vi "ScanSystemInfo.vi"(0 "refnum":refnum<file>, 11 "offset":i32) -> (1 "Scan Settings":T1 {"prf (kHz)" format="%.2f"; "GAIN(db)" items=["26.0", "40.0", "54.0"]; "LP FILT(IN MHz)" items=["20", "50", "100", "200"]; "HP FILT(IN KHz)" items=["1", "1000", "3000", "10000"]; "DAMPING (IN Ohm)" items=["7", "10", "16", "20", "26", "30", "40", "50"]; "ENERGY(UJ)" items=["1", "2", "4", "8", "16", "32"]}, 2 "Energy":u8, 3 "Damping":u8, 4 "dup refnum":refnum<file>, 6 "High Pass":u8, 8 "Gain":u8, 10 "prf (kHz)":sgl format="%.2f", 14 "Distance between\nscan planes (mm)":u16, 15 "Distance between\nscan lines (mm)":u16)   [LabVIEW 2022 SP3]
panel:
  out "Low Pass":u8
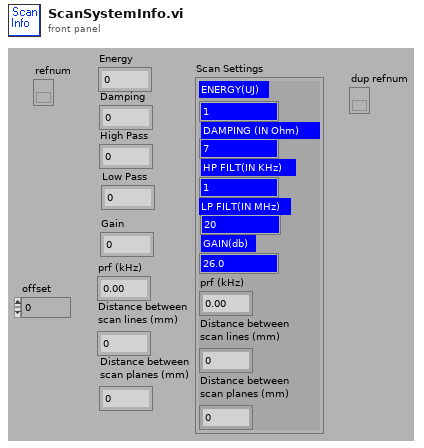
[diagram p1: front panel]
types:
  T1 = cluster{"ENERGY(UJ)":u8, "DAMPING (IN Ohm)":u8, "HP FILT(IN KHz) ":u8, "LP FILT(IN MHz)":u8, "GAIN(db)":u8, "prf (kHz)":sgl, "Distance between\nscan lines (mm)":u16, "Distance between\nscan planes (mm)":u16}
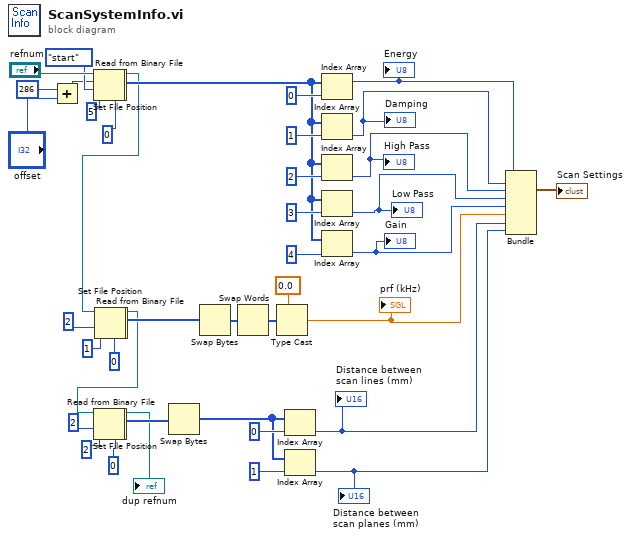
[diagram p0: block diagram]
diagram:
  n1 = Add(x=286 ("pos offset (0)"), y="offset") -> (x+y=w9:i32)
  n2 = Set File Position(offset (in bytes) (0)=w9, refnum="refnum", from (0:start)=enum16{"start", "end", "current"}."start" ("pos mode (0:2)")) -> (refnum out=w2:refnum<file>, error out=w1:errorcluster)  [unwired: 1 in]
  n3 = Read from Binary File(5:u8 0, 8:w1, 10:5 ("count"), 11:w2) -> (2:w26:u8[], 3:w25:refnum<file>)  [unwired: 4 out]
  n4 = Set File Position(refnum=w25, from (0:start)=2) -> (refnum out=w6:refnum<file>, error out=w5:errorcluster)  [unwired: 1 in, 1 out]
  n5 = Read from Binary File(5:0 ("byte stream type"), 8:w5, 10:1 ("count"), 11:w6) -> (2:w29:i32[], 3:w20:refnum<file>)  [unwired: 4 out]
  n6 = Set File Position(refnum=w20, from (0:start)=2) -> (refnum out=w4:refnum<file>, error out=w3:errorcluster)  [unwired: 1 in, 1 out]
  n7 = Read from Binary File(5:u16 0, 8:w3, 10:2 ("count"), 11:w4) -> (2:w17:u16[], 3:→"dup refnum":refnum<file>)  [unwired: 4 out]
  n8 = Swap Bytes(anything=w17) -> (byte swapped=w14:u16[])
  n9 = Swap Bytes(anything=w29) -> (byte swapped=w28:i32[])
  n10 = Swap Words(1:w28) -> (0:w27:i32[])
  n11 = Type Cast(type=sgl 0.0, x=w27) -> (*(type *) &x=w21:sgl)
  "prf (kHz)" <- w21
  n12 = Index Array(array=w14, index=0) -> (element=w13:u16)
  "Distance between\nscan lines (mm)" <- w13
  n13 = Index Array(array=w14, index=1) -> (element=w12:u16)
  "Distance between\nscan planes (mm)" <- w12
  n14 = Index Array(array=w26, index=0) -> (element=w34:u8)
  "Energy" <- w34
  n15 = Index Array(array=w26, index=1) -> (element=w33:u8)
  "Damping" <- w33
  n16 = Index Array(array=w26, index=2) -> (element=w32:u8)
  "High Pass" <- w32
  n17 = Index Array(array=w26, index=3) -> (element=w31:u8)
  "Low Pass" <- w31
  n18 = Index Array(array=w26, index=4) -> (element=w30:u8)
  "Gain" <- w30
  n19 = Bundle(w34, w33, w32, w31, w30, w21, w13, w12) -> (→"Scan Settings":cluster{u8, u8, u8, u8, u8, sgl, u16, u16})  [unwired: 1 out]
